vi "Read configuration.vi"(8 "error in":errorcluster, 11 "SystemLin Tag Module editor node in":refnum<class "SystemLin Tag Module editor node.lvclass">) -> (0 "error out":errorcluster, 2 "configuration":refnum<class "NISE_CEF_serializable configuration.lvclass">, 3 "SystemLin Tag Module editor node out":refnum<class "SystemLin Tag Module editor node.lvclass">)   [LabVIEW 2014, in "SystemLin Tag Module editor node.lvclass"]
uses:
  SystemLin Tag Module editor node.lvclass
  <vilib>/NI/Configuration Framework/serializable configuration/NISE_CEF_serializable configuration.lvclass
  SystemLin Tag Module editor node.lvclass/SystemLin Tag Module editor node.ctl
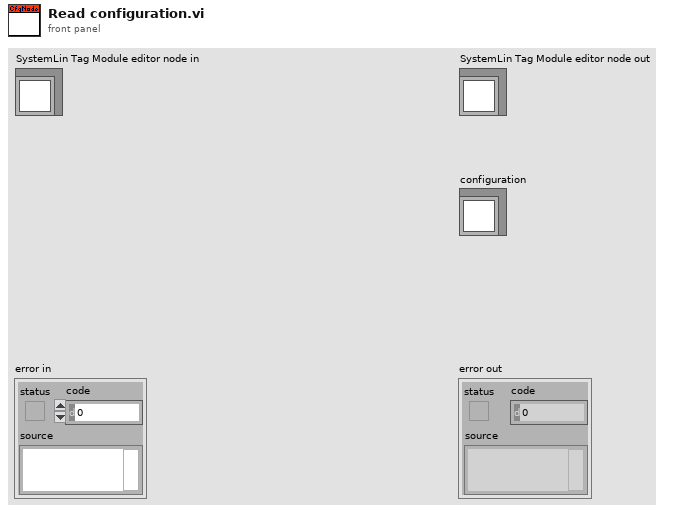
[diagram p1: front panel]
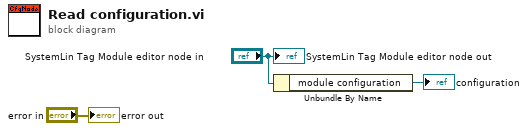
[diagram p0: block diagram]
diagram:
  n1 = Unbundle By Name("SystemLin Tag Module editor node in") -> ("module configuration"=→"configuration":refnum<class "SystemLin Tag Module configuration.lvclass">)
  "error out" <- "error in"
  "SystemLin Tag Module editor node out" <- "SystemLin Tag Module editor node in"
